vi "AirForceBalance.vi"(0 "Velocity (m/s)":dbl, 1 "Density (kg/m^3)":dbl, 2 "Numeric 5":dbl, 3 "NDHX XSection Area (m^2)":dbl, 4 "Velocity (m/s) 2":dbl, 5 "Density (kg/m^3) 2":dbl, 6 "Average":dbl, 8 "Stack Height (m)":dbl, 9 "Number Tube Rows":dbl, 10 "Louver Position (% Open)":dbl, 11 "Numeric 4":dbl, 12 "Friction Factor 2":dbl, 13 "Numeric 3":dbl, 14 "Friction Factor":dbl, 16 "Thermal Driving Force (Pa)":dbl) -> (18 "Louver Loss (Pa)":dbl, 20 "Wall Loss (Pa)":dbl, 21 "Louver K":dbl, 22 "Air Mass Acceleration (kg/s^2)":dbl, 23 "Exit Loss (Pa)":dbl, 24 "Turning Loss (Pa)":dbl, 25 "Bundle Loss (Pa)":dbl)   [LabVIEW 2019]
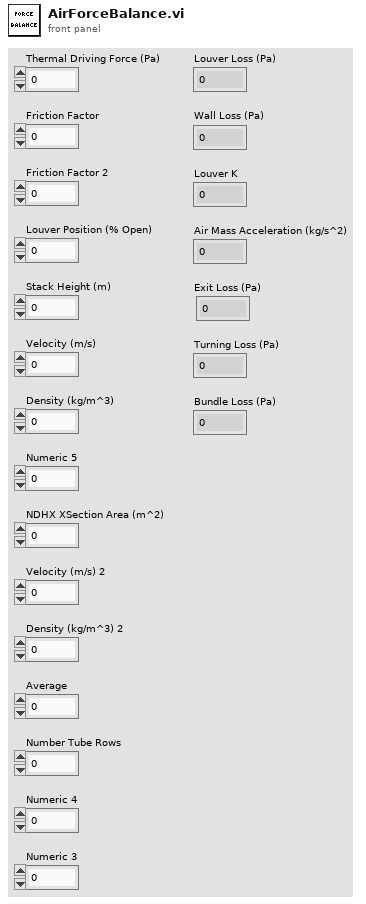
[diagram p1: front panel]
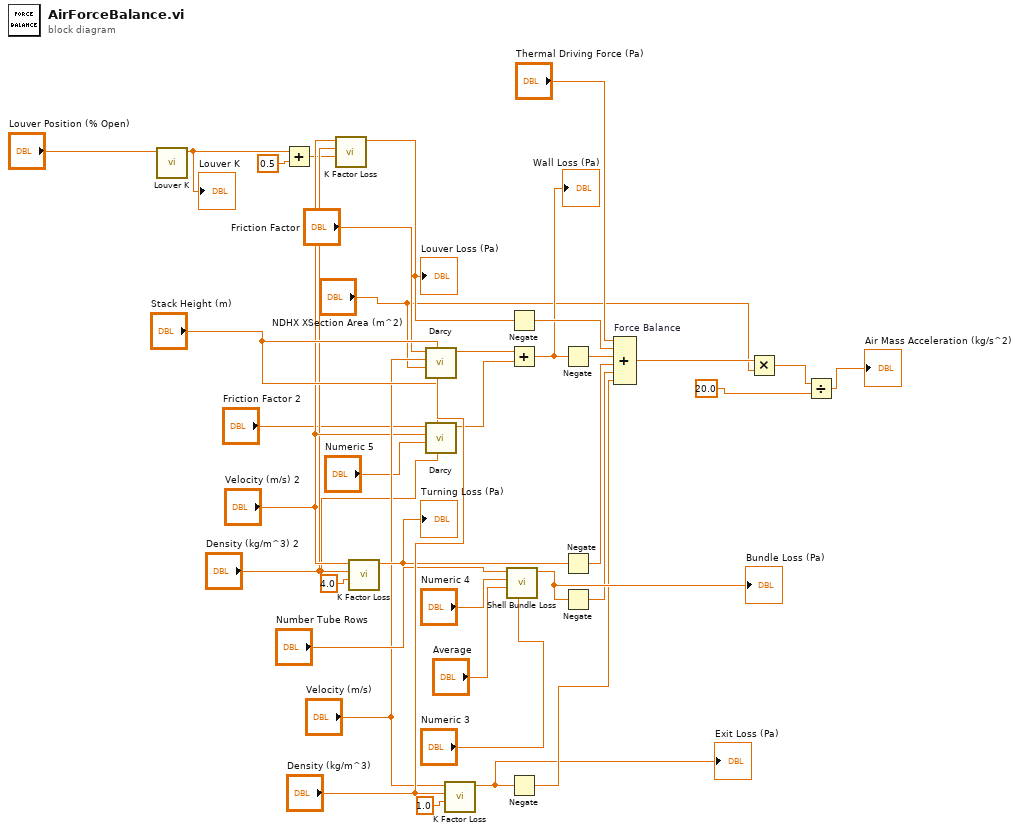
[diagram p0: block diagram]
diagram:
  n1 = call "Louver K.vi"("Louver Position"="Louver Position (% Open)") -> ("K"=w7:dbl)  [unwired: 10 in]
  "Louver K" <- w7
  n2 = Add(x=w7, y=0.5) -> (x+y=w8:dbl)
  n3 = call "K Factor Loss.vi"("K"=w8, "Density (kg/m^3)"="Density (kg/m^3) 2", "Velocity (m/s)"="Velocity (m/s) 2") -> ("Loss (Pa)"=w27:dbl)  [unwired: 8 in]
  "Louver Loss (Pa)" <- w27
  n4 = call "K Factor Loss.vi"("K"=4.0, "Density (kg/m^3)"="Density (kg/m^3) 2", "Velocity (m/s)"="Velocity (m/s) 2") -> ("Loss (Pa)"=w29:dbl)  [unwired: 8 in]
  "Turning Loss (Pa)" <- w29
  n5 = call "Darcy.vi"("Density (kg/m^3)"="Density (kg/m^3)", "Length (m)"="Stack Height (m)", "Effective Diameter (m)"="NDHX XSection Area (m^2)", "Velocity (m/s)"="Velocity (m/s)", "Friction Factor"="Friction Factor") -> ("Loss (Pa)"=w17:dbl)  [unwired: 6 in]
  n6 = call "Darcy.vi"("Density (kg/m^3)"="Density (kg/m^3) 2", "Length (m)"="Stack Height (m)", "Effective Diameter (m)"="Numeric 5", "Velocity (m/s)"="Velocity (m/s) 2", "Friction Factor"="Friction Factor 2") -> ("Loss (Pa)"=w18:dbl)  [unwired: 6 in]
  n7 = call "K Factor Loss.vi"("K"=1.0, "Density (kg/m^3)"="Density (kg/m^3)", "Velocity (m/s)"="Velocity (m/s)") -> ("Loss (Pa)"=w32:dbl)  [unwired: 8 in]
  "Exit Loss (Pa)" <- w32
  n8 = call "Shell Bundle Loss.vi"("Mass Flux (kg/s-m^2)"="Numeric 3", "Density (kg/m^3)"="Average", "Friction Factor"="Numeric 4", "Number Tube Rows"="Number Tube Rows") -> ("Bundle Loss (Pa)"=w36:dbl)  [unwired: 7 in]
  "Bundle Loss (Pa)" <- w36
  n9 = Negate(x=w27) -> (-x=w28:dbl)
  n10 = Add(x=w17, y=w18) -> (x+y=w24:dbl)
  "Wall Loss (Pa)" <- w24
  n11 = Negate(x=w32) -> (-x=w33:dbl)
  n12 = Negate(x=w24) -> (-x=w25:dbl)
  n13 = Negate(x=w29) -> (-x=w30:dbl)
  n14 = Negate(x=w36) -> (-x=w31:dbl)
  n15 = Compound Arithmetic op=ADD "Force Balance"("Thermal Driving Force (Pa)", w28, w25, w30, w31, w33) -> (w26:dbl)
  n16 = Multiply(x=w26, y="NDHX XSection Area (m^2)") -> (x*y=w2:dbl)
  n17 = Divide(x=w2, y=20.0) -> (x/y=→"Air Mass Acceleration (kg/s^2)":dbl)
